vi "Lab Panel V5.12.vi"() -> ()   [LabVIEW 2013] (continued)
                      tunnel: w5308 -> [w5324 _]
                      tunnel: [w5323 FALSE] -> w5291
                      frame False {
                        n2899 = Equal?(x=w5325, y=w5324) -> (x = y?=w5323:bool)
                      }
                      frame True {
                      }
                    }
                    n2900 = Or(x=w5292, y=w5291) -> (x .or. y?=w5286:bool)
                    n2901 = Or(x=w5290, y=w5289) -> (x .or. y?=w5285:bool)
                    n2902 = Or(x=w5293, y=w5294) -> (x .or. y?=w5281:bool)
                    n2903 = Or(x=w5286, y=w5285) -> (x .or. y?=w5284:bool)
                    n2904 = Or(x=w5283, y=w5284) -> (x .or. y?=w5282:bool)
                    n2905 = Or(x=w5282, y=w5281) -> (x .or. y?=w5280:bool)
                  }
                  frame #3 {
                    n2906 = local read "on loops"() -> (w5363:dbl)
                    n2907 = local read "jig cycle"() -> (w5360:dbl)
                    n2908 = local read "Send Mail Now"() -> (w5354:bool)
                    n2909 = Add(x=w5363, y=3.0) -> (x+y=w5361:dbl)
                    n2910 = Equal?(x=w5360, y=w5361) -> (x = y?=w5355:bool)
                    n2911 = And(x=w5355, y=w5354) -> (x .and. y?=w5353:bool)
                    n2912 = And(x=w5359, y=w5355) -> (x .and. y?=w5358:bool)
                    n2913 = And(x=w5358, y=w5357) -> (x .and. y?=w5356:bool)
                    n2914 = Or(x=w5356, y=w5353) -> (x .or. y?=w5352:bool)
                    n2915 = case shown="True" w5352 {
                      tunnel: w5368 -> [_ w5374]
                      tunnel: w5367 -> [_ w5373]
                      tunnel: "Lab Panel Test Status" -> [_ w5372]
                      tunnel: w5365 -> [_ w5371]
                      tunnel: w5364 -> [_ w5370]
                      tunnel: w5351 -> [_ w5369]
                      frame False {
                      }
                      frame True {
                        n2916 = stacked-sequence {
                          tunnel: w5374 -> [w5382 _]
                          tunnel: w5373 -> [w5381 _]
                          tunnel: w5372 -> [w5380 _]
                          tunnel: w5371 -> [w5379 _]
                          tunnel: w5370 -> [w5378 _]
                          tunnel: w5369 -> [w5377 _]
                          frame #0 {
                            n2917 = call "sub vi - send mail v5.vi"("TO:"=w5382, "subject"=w5380, "from"=w5378, "out going server"=w5379, "message"=w5381) -> ("error out"=w5376:errorcluster)  [unwired: 10 in]
                            n2918 = Bundle(cluster=w5377, "mail error"=w5376) -> (w5375:T7)  [unwired: 6 in]
                            n2919 = local write "MAIL SETTINGS"(w5375) -> ()
                          }
                          frame #1 {
                            n2920 = local write "mail control"("") -> ()
                            n2921 = local write "Send Mail Now"(FALSE) -> ()
                          }
                        }
                      }
                    }
                  }
                }
              }
            }
          }
          frame #18 {
            # "save jig cycle values once all run switches are off"
            n2922 = stacked-sequence {
              tunnel: w5394 -> [_ w5423]
              tunnel: w5393 -> [_ w5422]
              tunnel: w5392 -> [_ w5421]
              tunnel: w5391 -> [_ w5420]
              tunnel: w5390 -> [_ w5419]
              tunnel: w5389 -> [_ w5418]
              tunnel: w5388 -> [_ w5417]
              tunnel: w5387 -> [_ w5416]
              tunnel: w5386 -> [_ w5415]
              tunnel: w5385 -> [_ w5414]
              frame #0 {
              }
              frame #1 {
                n2923 = Not(x=w5414) -> (.not. x?=w5397:bool)
                n2924 = Not(x=w5422) -> (.not. x?=w5412:bool)
                n2925 = Not(x=w5419) -> (.not. x?=w5407:bool)
                n2926 = Not(x=w5417) -> (.not. x?=w5403:bool)
                n2927 = Not(x=w5415) -> (.not. x?=w5399:bool)
                n2928 = Not(x=w5423) -> (.not. x?=w5413:bool)
                n2929 = Not(x=w5421) -> (.not. x?=w5411:bool)
                n2930 = Not(x=w5418) -> (.not. x?=w5405:bool)
                n2931 = Not(x=w5420) -> (.not. x?=w5409:bool)
                n2932 = Not(x=w5416) -> (.not. x?=w5401:bool)
                n2933 = local read "Save JC"() -> (w5425:bool)
                n2934 = And(x=w5413, y=w5412) -> (x .and. y?=w5410:bool)
                n2935 = And(x=w5410, y=w5411) -> (x .and. y?=w5408:bool)
                n2936 = And(x=w5408, y=w5409) -> (x .and. y?=w5406:bool)
                n2937 = And(x=w5406, y=w5407) -> (x .and. y?=w5404:bool)
                n2938 = And(x=w5404, y=w5405) -> (x .and. y?=w5402:bool)
                n2939 = And(x=w5402, y=w5403) -> (x .and. y?=w5400:bool)
                n2940 = And(x=w5400, y=w5401) -> (x .and. y?=w5398:bool)
                n2941 = And(x=w5398, y=w5399) -> (x .and. y?=w5396:bool)
                n2942 = And(x=w5396, y=w5397) -> (x .and. y?=w5395:bool)
                n2943 = And(x=w5395, y=w5425) -> (x .and. y?=w5424:bool)
                n2944 = case shown="True" w5424 {
                  tunnel: w5395 -> [w5426 _]
                  frame False {
                    n2945 = case shown="False" w5426 {
                      frame False {
                        n2946 = local write "Save JC"(TRUE) -> ()
                      }
                      frame True {
                      }
                    }
                  }
                  frame True {
                    n2947 = stacked-sequence {
                      frame #0 {
                        n2948 = String To Path(string="c:\\crabtree\\Jig Cycles\\") -> (path=w5438:path)
                        n2949 = Build Path(base path=w5438, name or relative path="jigcycles.bin") -> (appended path=w5436:path)
                        n2950 = Create Folder(path (use dialog)=w5438) -> (error out=w5440:errorcluster)  [unwired: 2 in, 2 out]
                        n2951 = local read "JIG RELAY CYCLES"() -> (w5430:T8)
                        n2952 = call <vilib>:"Clear Errors.vi"("error in (no error)"=w5440) -> ()  [unwired: 6 in, 1 out]
                        n2953 = local write "Save JC"(FALSE) -> ()
                        n2954 = Open/Create/Replace File(file path (use dialog)=w5436, operation (0:open)=T21."replace or create") -> (refnum out=w5434:refnum<file>, error out=w5435:errorcluster)  [unwired: 4 in, 1 out]
                        n2955 = Write to Binary File(file (use dialog)=w5434, data=w5430, error in=w5435) -> (refnum out=w5433:refnum<file>, error out=w5432:errorcluster)  [unwired: 3 in, 1 out]
                        n2956 = Close File(refnum=w5433, error in=w5432) -> (error out=w5431:errorcluster)  [unwired: 1 out]
                        n2957 = local write "data file error"(w5431) -> ()
                      }
                      frame #1 {
                        n2958 = local read "JIG RELAY CYCLES"() -> (w5463:T8)
                        n2959 = Unbundle By Name(w5463) -> ("LAB01-1"=w5458:dbl, "LAB01-2"=w5457:dbl, "LAB02-1"=w5455:dbl, "LAB02-2"=w5454:dbl, "LAB03-1"=w5452:dbl, "LAB03-2"=w5449:dbl, "LAB04-1"=w5448:dbl, "LAB04-2"=w5446:dbl, "LAB05-1"=w5444:dbl, "LAB05-2"=w5442:dbl)
                        n2960 = stacked-sequence {
                          tunnel: w5458 -> [w5466 _ _ _ _ _ _ _ _ _]
                          tunnel: 1000000 -> [w5469 w5479 w5489 w5499 w5509 w5519 w5529 w5539 w5549 w5559]
                          tunnel: [w5467 _ _ _ _ _ _ _ _ _] -> w5461
                          tunnel: "TEST STATION HAS REACHED 1 MILLION CYCLES, REPLACE  CONTROL RELAYS" -> [w5465 w5477 w5487 w5497 w5507 w5517 w5527 w5537 w5547 w5557]
                          tunnel: [_ w5476 _ _ _ _ _ _ _ _] -> w5459
                          tunnel: w5457 -> [_ w5475 _ _ _ _ _ _ _ _]
                          tunnel: [_ _ w5486 _ _ _ _ _ _ _] -> w5456
                          tunnel: w5455 -> [_ _ w5485 _ _ _ _ _ _ _]
                          tunnel: w5454 -> [_ _ _ w5496 _ _ _ _ _ _]
                          tunnel: [_ _ _ w5495 _ _ _ _ _ _] -> w5453
                          tunnel: w5452 -> [_ _ _ _ w5506 _ _ _ _ _]
                          tunnel: [_ _ _ _ w5505 _ _ _ _ _] -> w5451
                          tunnel: [_ _ _ _ _ w5516 _ _ _ _] -> w5450
                          tunnel: w5449 -> [_ _ _ _ _ w5515 _ _ _ _]
                          tunnel: w5448 -> [_ _ _ _ _ _ w5526 _ _ _]
                          tunnel: [_ _ _ _ _ _ w5525 _ _ _] -> w5447
                          tunnel: w5446 -> [_ _ _ _ _ _ _ w5536 _ _]
                          tunnel: [_ _ _ _ _ _ _ w5535 _ _] -> w5445
                          tunnel: w5444 -> [_ _ _ _ _ _ _ _ w5546 _]
                          tunnel: [_ _ _ _ _ _ _ _ w5545 _] -> w5443
                          tunnel: w5442 -> [_ _ _ _ _ _ _ _ _ w5556]
                          tunnel: [_ _ _ _ _ _ _ _ _ w5555] -> w5441
                          frame #0 {
                            n2961 = Greater?(x=w5466, y=w5469) -> (0:w5468:bool)
                            n2962 = case shown="True" w5468 {
                              tunnel: [w5470 0] -> w5467
                              tunnel: w5466 -> [w5470 _]
                              tunnel: w5465 -> [_ w5471]
                              frame False {
                              }
                              frame True {
                                n2963 = Concatenate Strings("LA01-1 ", w5471) -> (w5474:string)
                                n2964 = One Button Dialog(message=w5474) -> ()  [unwired: 1 in, 1 out]
                              }
                            }
                          }
                          frame #1 {
                            n2965 = Greater?(x=w5475, y=w5479) -> (0:w5478:bool)
                            n2966 = case shown="True" w5478 {
                              tunnel: [w5480 0] -> w5476
                              tunnel: w5475 -> [w5480 _]
                              tunnel: w5477 -> [_ w5481]
                              frame False {
                              }
                              frame True {
                                n2967 = Concatenate Strings("LA01-2 ", w5481) -> (w5484:string)
                                n2968 = One Button Dialog(message=w5484) -> ()  [unwired: 1 in, 1 out]
                              }
                            }
                          }
                          frame #2 {
                            n2969 = Greater?(x=w5485, y=w5489) -> (0:w5488:bool)
                            n2970 = case shown="True" w5488 {
                              tunnel: [w5490 0] -> w5486
                              tunnel: w5485 -> [w5490 _]
                              tunnel: w5487 -> [_ w5491]
                              frame False {
                              }
                              frame True {
                                n2971 = Concatenate Strings("LA02-1 ", w5491) -> (w5494:string)
                                n2972 = One Button Dialog(message=w5494) -> ()  [unwired: 1 in, 1 out]
                              }
                            }
                          }
                          frame #3 {
                            n2973 = Greater?(x=w5496, y=w5499) -> (0:w5498:bool)
                            n2974 = case shown="True" w5498 {
                              tunnel: [w5500 0] -> w5495
                              tunnel: w5496 -> [w5500 _]
                              tunnel: w5497 -> [_ w5501]
                              frame False {
                              }
                              frame True {
                                n2975 = Concatenate Strings("LA02-2 ", w5501) -> (w5504:string)
                                n2976 = One Button Dialog(message=w5504) -> ()  [unwired: 1 in, 1 out]
                              }
                            }
                          }
                          frame #4 {
                            n2977 = Greater?(x=w5506, y=w5509) -> (0:w5508:bool)
                            n2978 = case shown="True" w5508 {
                              tunnel: [w5510 0] -> w5505
                              tunnel: w5506 -> [w5510 _]
                              tunnel: w5507 -> [_ w5511]
                              frame False {
                              }
                              frame True {
                                n2979 = Concatenate Strings("LA03-1 ", w5511) -> (w5514:string)
                                n2980 = One Button Dialog(message=w5514) -> ()  [unwired: 1 in, 1 out]
                              }
                            }
                          }
                          frame #5 {
                            n2981 = Greater?(x=w5515, y=w5519) -> (0:w5518:bool)
                            n2982 = case shown="True" w5518 {
                              tunnel: [w5520 0] -> w5516
                              tunnel: w5515 -> [w5520 _]
                              tunnel: w5517 -> [_ w5521]
                              frame False {
                              }
                              frame True {
                                n2983 = Concatenate Strings("LA03-2 ", w5521) -> (w5524:string)
                                n2984 = One Button Dialog(message=w5524) -> ()  [unwired: 1 in, 1 out]
                              }
                            }
                          }
                          frame #6 {
                            n2985 = Greater?(x=w5526, y=w5529) -> (0:w5528:bool)
                            n2986 = case shown="True" w5528 {
                              tunnel: [w5530 0] -> w5525
                              tunnel: w5526 -> [w5530 _]
                              tunnel: w5527 -> [_ w5531]
                              frame False {
                              }
                              frame True {
                                n2987 = Concatenate Strings("LA04-1 ", w5531) -> (w5534:string)
                                n2988 = One Button Dialog(message=w5534) -> ()  [unwired: 1 in, 1 out]
                              }
                            }
                          }
                          frame #7 {
                            n2989 = Greater?(x=w5536, y=w5539) -> (0:w5538:bool)
                            n2990 = case shown="True" w5538 {
                              tunnel: [w5540 0] -> w5535
                              tunnel: w5536 -> [w5540 _]
                              tunnel: w5537 -> [_ w5541]
                              frame False {
                              }
                              frame True {
                                n2991 = Concatenate Strings("LA04-2 ", w5541) -> (w5544:string)
                                n2992 = One Button Dialog(message=w5544) -> ()  [unwired: 1 in, 1 out]
                              }
                            }
                          }
                          frame #8 {
                            n2993 = Greater?(x=w5546, y=w5549) -> (0:w5548:bool)
                            n2994 = case shown="True" w5548 {
                              tunnel: [w5550 0] -> w5545
                              tunnel: w5546 -> [w5550 _]
                              tunnel: w5547 -> [_ w5551]
                              frame False {
                              }
                              frame True {
                                n2995 = Concatenate Strings("LA05-1 ", w5551) -> (w5554:string)
                                n2996 = One Button Dialog(message=w5554) -> ()  [unwired: 1 in, 1 out]
                              }
                            }
                          }
                          frame #9 {
                            n2997 = Greater?(x=w5556, y=w5559) -> (0:w5558:bool)
                            n2998 = case shown="True" w5558 {
                              tunnel: [w5560 0] -> w5555
                              tunnel: w5556 -> [w5560 _]
                              tunnel: w5557 -> [_ w5561]
                              frame False {
                              }
                              frame True {
                                n2999 = Concatenate Strings("LA05-2 ", w5561) -> (w5564:string)
                                n3000 = One Button Dialog(message=w5564) -> ()  [unwired: 1 in, 1 out]
                              }
                            }
                          }
                        }
                        n3001 = Bundle By Name(cluster=w5463, "LAB01-1"=w5461, "LAB01-2"=w5459, "LAB02-1"=w5456, "LAB02-2"=w5453, "LAB03-1"=w5451, "LAB03-2"=w5450, "LAB04-1"=w5447, "LAB04-2"=w5445, "LAB05-1"=w5443, "LAB05-2"=w5441) -> (w5462:T8)
                        n3002 = local write "JIG RELAY CYCLES"(w5462) -> ()
                      }
                    }
                  }
                }
              }
            }
          }
          frame #19 {
            # "get temperature values"
            n3003 = local read "Panel #"() -> (w5565:dbl)
            n3004 = local read "Simulate"() -> (w5578:bool)
            n3005 = local read "Temp Test Cal"() -> (w5575:dbl)
            n3006 = stacked-sequence {
              seq-local: [w5581 _] -> [_ w5624]
              tunnel: w5578 -> [_ w5638]
              tunnel: T14 {"1  (A) cal"=1.0, "1 (V) cal"=1.0, "1 (PF) cal"=1.0, "1 (TL) cal"=1.0, "1 (TN) cal"=1.0, "2 (A) cal"=1.0, "2 (V) cal"=1.0, "2 (PF) cal"=1.0, "2 (TL) cal"=1.0, "2 (TN) cal"=1.0} ("CAL LAB01") -> [_ w5637]
              tunnel: w5576 -> [_ w5636]
              tunnel: w5575 -> [_ w5635]
              tunnel: w5574 -> [_ w5634]
              tunnel: w5573 -> [_ w5633]
              tunnel: w5572 -> [_ w5632]
              tunnel: w5571 -> [_ w5631]
              tunnel: w5570 -> [_ w5630]
              tunnel: w5569 -> [_ w5629]
              tunnel: w5568 -> [_ w5628]
              tunnel: w5567 -> [_ w5627]
              tunnel: w5566 -> [_ w5626]
              tunnel: w5565 -> [_ w5625]
              frame #0 {
                n3007 = local read "Select COM port"() -> (w5582:refnum<visa-resource-name>)
                "COM port" <- w5582
                n3008 = global write "Global 1.vi" "COM port"(w5582) -> ()
                n3009 = global write "Global 1.vi" "tmp dly lps"("Temp Delay Lps") -> ()
                n3010 = global write "Global 1.vi" "dly value"("Temp Value") -> ()
                n3011 = local read "jig cycle"() -> (w5584:dbl)
                n3012 = local read "on loops"() -> (w5586:dbl)
                n3013 = Add(x=w5586, y=3) -> (x+y=w5587:dbl)
                n3014 = local read "Panel #"() -> (w5583:dbl)
                n3015 = Equal?(x=w5584, y=w5587) -> (x = y?=w5581:bool)
                n3016 = case shown="True" w5581 {
                  tunnel: w5583 -> [_ w5592]
                  frame False {
                  }
                  frame True {
                    n3017 = local read "Simulate"() -> (w5589:bool)
                    n3018 = case shown="1" w5592 {
                      tunnel: 1.0 -> [_ w5599 w5602 w5609 w5614 w5620]
                      tunnel: w5589 -> [_ w5595 w5601 w5607 w5615 w5619]
                      tunnel: [FALSE w5594 w5600 w5606 w5612 w5618] -> w5588
                      frame 0, Default {
                      }
                      frame 1 {
                        w5597 = FALSE
                        n3019 = call "sub vi - GET ALL TEMP v7.vi"("LA01-EN"=TRUE, "simulate"=w5595, "LA02-EN"=w5597, "LA03-EN"=w5597, "LA04-EN"=w5597, "LA05-EN"=w5597, "Gen Cal Value"=w5599) -> ("LA01 TEMP"=w5596:T24, "error"=w5594:bool)  [unwired: 3 in, 4 out]
                        n3020 = local write "LAB01 TEMP"(w5596) -> ()
                      }
                      frame 2 {
                        w5603 = FALSE
                        n3021 = call "sub vi - GET ALL TEMP v7.vi"("LA01-EN"=w5603, "simulate"=w5601, "LA02-EN"=TRUE, "LA03-EN"=w5603, "LA04-EN"=w5603, "LA05-EN"=w5603, "Gen Cal Value"=w5602) -> ("LA02 TEMP"=w5605:T24, "error"=w5600:bool)  [unwired: 3 in, 4 out]
                        n3022 = local write "LAB02 TEMP"(w5605) -> ()
                      }
                      frame 3 {
                        w5610 = FALSE
                        n3023 = call "sub vi - GET ALL TEMP v7.vi"("LA01-EN"=w5610, "simulate"=w5607, "LA02-EN"=w5610, "LA03-EN"=TRUE, "LA04-EN"=w5610, "LA05-EN"=w5610, "Gen Cal Value"=w5609) -> ("LA03 TEMP"=w5608:T24, "error"=w5606:bool)  [unwired: 3 in, 4 out]
                        n3024 = local write "LAB03 TEMP"(w5608) -> ()
                      }
                      frame 4 {
                        w5616 = FALSE
                        n3025 = call "sub vi - GET ALL TEMP v7.vi"("LA01-EN"=w5616, "simulate"=w5615, "LA02-EN"=w5616, "LA03-EN"=w5616, "LA04-EN"=TRUE, "LA05-EN"=w5616, "Gen Cal Value"=w5614) -> ("LA04 TEMP"=w5613:T24, "error"=w5612:bool)  [unwired: 3 in, 4 out]
                        n3026 = local write "LAB04 TEMP"(w5613) -> ()
                      }
                      frame 5 {
                        w5622 = FALSE
                        n3027 = call "sub vi - GET ALL TEMP v7.vi"("LA01-EN"=w5622, "simulate"=w5619, "LA02-EN"=w5622, "LA03-EN"=w5622, "LA04-EN"=w5622, "LA05-EN"=TRUE, "Gen Cal Value"=w5620) -> ("error"=w5618:bool, "LA05 TEMP"=w5621:T24)  [unwired: 3 in, 4 out]
                        n3028 = local write "LAB05 TEMP"(w5621) -> ()
                      }
                    }
                    "Error Temp" <- w5588
                    n3029 = local write "TEMP"(TRUE) -> ()
                  }
                }
              }
              frame #1 {
                n3030 = case shown="True" w5624 {
                  tunnel: w5638 -> [_ w5652]
                  tunnel: w5637 -> [_ w5651]
                  tunnel: w5636 -> [_ w5650]
                  tunnel: w5635 -> [_ w5649]
                  tunnel: w5634 -> [_ w5648]
                  tunnel: w5633 -> [_ w5647]
                  tunnel: w5632 -> [_ w5646]
                  tunnel: w5631 -> [_ w5645]
                  tunnel: w5630 -> [_ w5644]
                  tunnel: w5629 -> [_ w5643]
                  tunnel: w5628 -> [_ w5642]
                  tunnel: w5627 -> [_ w5641]
                  tunnel: w5626 -> [_ w5640]
                  tunnel: w5625 -> [_ w5639]
                  frame False {
                  }
                  frame True {
                    n3031 = case shown="1" w5639 {
                      tunnel: w5652 -> [_ w5665 w5710 w5755 w5800 w5845]
                      tunnel: w5651 -> [_ w5664 w5709 w5754 w5799 w5844]
                      tunnel: w5650 -> [_ w5654 _ _ _ _]
                      tunnel: w5649 -> [_ w5659 w5708 w5753 w5798 w5843]
                      tunnel: w5648 -> [_ w5653 _ _ _ _]
                      tunnel: w5647 -> [_ _ w5699 _ _ _]
                      tunnel: w5646 -> [_ _ w5698 _ _ _]
                      tunnel: w5645 -> [_ _ _ w5744 _ _]
                      tunnel: w5644 -> [_ _ _ w5743 _ _]
                      tunnel: w5643 -> [_ _ _ _ w5789 _]
                      tunnel: w5642 -> [_ _ _ _ w5788 _]
                      tunnel: w5641 -> [_ _ _ _ _ w5834]
                      tunnel: w5640 -> [_ _ _ _ _ w5833]
                      frame ..0 {
                      }
                      frame 1 {
                        n3032 = case shown="False" w5665 {
                          tunnel: [w5696 w5697] -> w5681
                          tunnel: w5664 -> [_ w5697]
                          frame False {
                            n3033 = local read "CAL LAB01"() -> (w5696:T14)
                          }
                          frame True {
                          }
                        }
                        n3034 = local read "TEMP LA01"() -> (w5672:T9)
                        n3035 = local read "LAB01 TEMP"() -> (w5671:T12)
                        n3036 = call "sub vi - temperature delay v3.vi"("2-run"=w5653, "1-run"=w5654, "temp values IN"=w5672, "temp signals"=w5671) -> ("T2-N"=w5667:dbl, "T2-L"=w5668:dbl, "T1-N"=w5669:dbl, "T1-L"=w5670:dbl, "temp values OUT"=w5666:T43)  [unwired: 3 in]
                        n3037 = Unbundle By Name(w5681) -> ("1 (TL) cal"=w5676:dbl, "1 (TN) cal"=w5675:dbl, "2 (TL) cal"=w5674:dbl, "2 (TN) cal"=w5673:dbl)  [unwired: 6 out]
                        n3038 = local write "TEMP LA01"(w5666) -> ()
                        n3039 = Multiply(x=w5670, y=w5676) -> (x*y=w5663:dbl)
                        n3040 = Multiply(x=w5669, y=w5675) -> (x*y=w5661:dbl)
                        n3041 = Multiply(x=w5668, y=w5674) -> (x*y=w5658:dbl)
                        n3042 = Multiply(x=w5667, y=w5673) -> (x*y=w5657:dbl)
                        n3043 = case shown="True" w5654 {
                          tunnel: w5663 -> [w5690 w5695]
                          tunnel: w5659 -> [_ w5693]
                          tunnel: [w5690 w5694] -> w5662
                          tunnel: w5661 -> [w5689 w5692]
                          tunnel: [w5689 w5691] -> w5660
                          frame False {
                          }
                          frame True {
                            n3044 = Multiply(x=w5693, y=w5692) -> (x*y=w5691:dbl)
                            n3045 = Multiply(x=w5693, y=w5695) -> (x*y=w5694:dbl)
                          }
                        }
                        n3046 = case shown="True" w5653 {
                          tunnel: w5658 -> [w5683 w5688]
                          tunnel: w5659 -> [_ w5686]
                          tunnel: [w5683 w5687] -> w5656
                          tunnel: w5657 -> [w5682 w5685]
                          tunnel: [w5682 w5684] -> w5655
                          frame False {
                          }
                          frame True {
                            n3047 = Multiply(x=w5686, y=w5685) -> (x*y=w5684:dbl)
                            n3048 = Multiply(x=w5686, y=w5688) -> (x*y=w5687:dbl)
                          }
                        }
                        n3049 = local read "SIG LAB01-2"() -> (w5678:T2)
                        n3050 = local read "SIG LAB01-1"() -> (w5680:T2)
                        n3051 = Bundle By Name(cluster=w5680, "Tmp Live"=w5662, "Tmp Neut"=w5660) -> (w5679:T2)
                        n3052 = Bundle By Name(cluster=w5678, "Tmp Live"=w5656, "Tmp Neut"=w5655) -> (w5677:T2)
                        n3053 = local write "SIG LAB01-1"(w5679) -> ()
                        n3054 = local write "SIG LAB01-2"(w5677) -> ()
                      }
                      frame 2 {
                        n3055 = case shown="True" w5710 {
                          tunnel: [w5741 w5742] -> w5726
                          tunnel: w5709 -> [_ w5742]
                          frame False {
                            n3056 = local read "CAL LAB02"() -> (w5741:T15)
                          }
                          frame True {
                          }
                        }
                        n3057 = local read "LAB02 TEMP"() -> (w5717:T12)
                        n3058 = local read "TEMP LA02"() -> (w5716:T9)
                        n3059 = call "sub vi - temperature delay v3.vi"("2-run"=w5698, "1-run"=w5699, "temp values IN"=w5716, "temp signals"=w5717) -> ("T2-N"=w5711:dbl, "T2-L"=w5712:dbl, "T1-N"=w5713:dbl, "T1-L"=w5714:dbl, "temp values OUT"=w5715:T43)  [unwired: 3 in]
                        n3060 = Unbundle By Name(w5726) -> ("1 (TL) cal"=w5721:dbl, "1 (TN) cal"=w5720:dbl, "2 (TL) cal"=w5719:dbl, "2 (TN) cal"=w5718:dbl)  [unwired: 6 out]
                        n3061 = local write "TEMP LA02"(w5715) -> ()
                        n3062 = Multiply(x=w5714, y=w5721) -> (x*y=w5707:dbl)
                        n3063 = Multiply(x=w5713, y=w5720) -> (x*y=w5706:dbl)
                        n3064 = Multiply(x=w5712, y=w5719) -> (x*y=w5703:dbl)
                        n3065 = Multiply(x=w5711, y=w5718) -> (x*y=w5702:dbl)
                        n3066 = case shown="True" w5699 {
                          tunnel: w5707 -> [w5735 w5740]
                          tunnel: w5708 -> [_ w5738]
                          tunnel: [w5735 w5739] -> w5705
                          tunnel: w5706 -> [w5734 w5737]
                          tunnel: [w5734 w5736] -> w5704
                          frame False {
                          }
                          frame True {
                            n3067 = Multiply(x=w5738, y=w5737) -> (x*y=w5736:dbl)
                            n3068 = Multiply(x=w5738, y=w5740) -> (x*y=w5739:dbl)
                          }
                        }
                        n3069 = case shown="True" w5698 {
                          tunnel: w5703 -> [w5728 w5733]
                          tunnel: w5708 -> [_ w5731]
                          tunnel: [w5728 w5732] -> w5701
                          tunnel: w5702 -> [w5727 w5730]
                          tunnel: [w5727 w5729] -> w5700
                          frame False {
                          }
                          frame True {
                            n3070 = Multiply(x=w5731, y=w5730) -> (x*y=w5729:dbl)
                            n3071 = Multiply(x=w5731, y=w5733) -> (x*y=w5732:dbl)
                          }
                        }
                        n3072 = local read "SIG LAB02-2"() -> (w5723:T2)
                        n3073 = local read "SIG LAB02-1"() -> (w5725:T2)
                        n3074 = Bundle By Name(cluster=w5725, "Tmp Live"=w5705, "Tmp Neut"=w5704) -> (w5724:T2)
                        n3075 = Bundle By Name(cluster=w5723, "Tmp Live"=w5701, "Tmp Neut"=w5700) -> (w5722:T2)
                        n3076 = local write "SIG LAB02-1"(w5724) -> ()
                        n3077 = local write "SIG LAB02-2"(w5722) -> ()
                      }
                      frame 3 {
                        n3078 = case shown="False" w5755 {
                          tunnel: [w5786 w5787] -> w5771
                          tunnel: w5754 -> [_ w5787]
                          frame False {
                            n3079 = local read "CAL LAB03"() -> (w5786:T14)
                          }
                          frame True {
                          }
                        }
                        n3080 = local read "TEMP LA03"() -> (w5761:T9)
                        n3081 = local read "LAB03 TEMP"() -> (w5762:T12)
                        n3082 = call "sub vi - temperature delay v3.vi"("2-run"=w5743, "1-run"=w5744, "temp values IN"=w5761, "temp signals"=w5762) -> ("T2-N"=w5756:dbl, "T2-L"=w5757:dbl, "T1-N"=w5758:dbl, "T1-L"=w5759:dbl, "temp values OUT"=w5760:T43)  [unwired: 3 in]
                        n3083 = Unbundle By Name(w5771) -> ("1 (TL) cal"=w5766:dbl, "1 (TN) cal"=w5765:dbl, "2 (TL) cal"=w5764:dbl, "2 (TN) cal"=w5763:dbl)  [unwired: 6 out]
                        n3084 = local write "TEMP LA03"(w5760) -> ()
                        n3085 = Multiply(x=w5759, y=w5766) -> (x*y=w5752:dbl)
                        n3086 = Multiply(x=w5758, y=w5765) -> (x*y=w5751:dbl)
                        n3087 = Multiply(x=w5757, y=w5764) -> (x*y=w5748:dbl)
                        n3088 = Multiply(x=w5756, y=w5763) -> (x*y=w5747:dbl)
                        n3089 = case shown="True" w5743 {
                          tunnel: w5748 -> [w5773 w5778]
                          tunnel: w5753 -> [_ w5776]
                          tunnel: [w5773 w5777] -> w5746
                          tunnel: w5747 -> [w5772 w5775]
                          tunnel: [w5772 w5774] -> w5745
                          frame False {
                          }
                          frame True {
                            n3090 = Multiply(x=w5776, y=w5775) -> (x*y=w5774:dbl)
                            n3091 = Multiply(x=w5776, y=w5778) -> (x*y=w5777:dbl)
                          }
                        }
                        n3092 = case shown="True" w5744 {
                          tunnel: w5752 -> [w5780 w5785]
                          tunnel: w5753 -> [_ w5783]
                          tunnel: [w5780 w5784] -> w5750
                          tunnel: w5751 -> [w5779 w5782]
                          tunnel: [w5779 w5781] -> w5749
                          frame False {
                          }
                          frame True {
                            n3093 = Multiply(x=w5783, y=w5782) -> (x*y=w5781:dbl)
                            n3094 = Multiply(x=w5783, y=w5785) -> (x*y=w5784:dbl)
                          }
                        }
                        n3095 = local read "SIG LAB03-2"() -> (w5768:T2)
                        n3096 = local read "SIG LAB03-1"() -> (w5770:T2)
                        n3097 = Bundle By Name(cluster=w5770, "Tmp Live"=w5750, "Tmp Neut"=w5749) -> (w5769:T2)
                        n3098 = Bundle By Name(cluster=w5768, "Tmp Live"=w5746, "Tmp Neut"=w5745) -> (w5767:T2)
                        n3099 = local write "SIG LAB03-1"(w5769) -> ()
                        n3100 = local write "SIG LAB03-2"(w5767) -> ()
                      }
                      frame 4 {
                        n3101 = case shown="False" w5800 {
                          tunnel: [w5831 w5832] -> w5816
                          tunnel: w5799 -> [_ w5832]
                          frame False {
                            n3102 = local read "CAL LAB04"() -> (w5831:T14)
                          }
                          frame True {
                          }
                        }
                        n3103 = local read "LAB04 TEMP"() -> (w5806:T12)
                        n3104 = local read "TEMP LA04"() -> (w5807:T9)
                        n3105 = call "sub vi - temperature delay v3.vi"("2-run"=w5788, "1-run"=w5789, "temp values IN"=w5807, "temp signals"=w5806) -> ("T2-N"=w5801:dbl, "T2-L"=w5802:dbl, "T1-N"=w5803:dbl, "T1-L"=w5804:dbl, "temp values OUT"=w5805:T43)  [unwired: 3 in]
                        n3106 = Unbundle By Name(w5816) -> ("1 (TL) cal"=w5811:dbl, "1 (TN) cal"=w5810:dbl, "2 (TL) cal"=w5809:dbl, "2 (TN) cal"=w5808:dbl)  [unwired: 6 out]
                        n3107 = local write "TEMP LA04"(w5805) -> ()
                        n3108 = Multiply(x=w5804, y=w5811) -> (x*y=w5797:dbl)
                        n3109 = Multiply(x=w5803, y=w5810) -> (x*y=w5796:dbl)
                        n3110 = Multiply(x=w5802, y=w5809) -> (x*y=w5793:dbl)
                        n3111 = Multiply(x=w5801, y=w5808) -> (x*y=w5792:dbl)
                        n3112 = case shown="True" w5788 {
                          tunnel: w5793 -> [w5818 w5823]
                          tunnel: w5798 -> [_ w5821]
                          tunnel: [w5818 w5822] -> w5791
                          tunnel: w5792 -> [w5817 w5820]
                          tunnel: [w5817 w5819] -> w5790
                          frame False {
                          }
                          frame True {
                            n3113 = Multiply(x=w5821, y=w5820) -> (x*y=w5819:dbl)
                            n3114 = Multiply(x=w5821, y=w5823) -> (x*y=w5822:dbl)
                          }
                        }
                        n3115 = case shown="True" w5789 {
                          tunnel: w5797 -> [w5825 w5830]
                          tunnel: w5798 -> [_ w5828]
                          tunnel: [w5825 w5829] -> w5795
                          tunnel: w5796 -> [w5824 w5827]
                          tunnel: [w5824 w5826] -> w5794
                          frame False {
                          }
                          frame True {
                            n3116 = Multiply(x=w5828, y=w5827) -> (x*y=w5826:dbl)
                            n3117 = Multiply(x=w5828, y=w5830) -> (x*y=w5829:dbl)
                          }
                        }
                        n3118 = local read "SIG LAB04-2"() -> (w5813:T2)
                        n3119 = local read "SIG LAB04-1"() -> (w5815:T2)
                        n3120 = Bundle By Name(cluster=w5815, "Tmp Live"=w5795, "Tmp Neut"=w5794) -> (w5814:T2)
                        n3121 = Bundle By Name(cluster=w5813, "Tmp Live"=w5791, "Tmp Neut"=w5790) -> (w5812:T2)
                        n3122 = local write "SIG LAB04-1"(w5814) -> ()
                        n3123 = local write "SIG LAB04-2"(w5812) -> ()
                      }
                      frame 5.. {
                        n3124 = case shown="False" w5845 {
                          tunnel: [w5876 w5877] -> w5861
                          tunnel: w5844 -> [_ w5877]
                          frame False {
                            n3125 = local read "CAL LAB05"() -> (w5876:T14)
                          }
                          frame True {
                          }
                        }
                        n3126 = local read "LAB05 TEMP"() -> (w5851:T12)
                        n3127 = local read "TEMP LA05"() -> (w5852:T9)
                        n3128 = call "sub vi - temperature delay v3.vi"("2-run"=w5833, "1-run"=w5834, "temp values IN"=w5852, "temp signals"=w5851) -> ("T2-N"=w5847:dbl, "T2-L"=w5848:dbl, "T1-N"=w5849:dbl, "T1-L"=w5850:dbl, "temp values OUT"=w5846:T43)  [unwired: 3 in]
                        n3129 = local write "TEMP LA05"(w5846) -> ()
                        n3130 = Unbundle By Name(w5861) -> ("1 (TL) cal"=w5853:dbl, "1 (TN) cal"=w5856:dbl, "2 (TL) cal"=w5855:dbl, "2 (TN) cal"=w5854:dbl)  [unwired: 6 out]
                        n3131 = Multiply(x=w5850, y=w5853) -> (x*y=w5842:dbl)
                        n3132 = Multiply(x=w5849, y=w5856) -> (x*y=w5841:dbl)
                        n3133 = Multiply(x=w5848, y=w5855) -> (x*y=w5838:dbl)
                        n3134 = Multiply(x=w5847, y=w5854) -> (x*y=w5837:dbl)
                        n3135 = case shown="True" w5833 {
                          tunnel: w5838 -> [w5863 w5868]
                          tunnel: w5843 -> [_ w5866]
                          tunnel: [w5863 w5867] -> w5836
                          tunnel: w5837 -> [w5862 w5865]
                          tunnel: [w5862 w5864] -> w5835
                          frame False {
                          }
                          frame True {
                            n3136 = Multiply(x=w5866, y=w5865) -> (x*y=w5864:dbl)
                            n3137 = Multiply(x=w5866, y=w5868) -> (x*y=w5867:dbl)
                          }
                        }
                        n3138 = case shown="True" w5834 {
                          tunnel: w5842 -> [w5870 w5875]
                          tunnel: w5843 -> [_ w5873]
                          tunnel: [w5870 w5874] -> w5840
                          tunnel: w5841 -> [w5869 w5872]
                          tunnel: [w5869 w5871] -> w5839
                          frame False {
                          }
                          frame True {
                            n3139 = Multiply(x=w5873, y=w5872) -> (x*y=w5871:dbl)
                            n3140 = Multiply(x=w5873, y=w5875) -> (x*y=w5874:dbl)
                          }
                        }
                        n3141 = local read "SIG LAB05-1"() -> (w5860:T2)
                        n3142 = Bundle By Name(cluster=w5860, "Tmp Live"=w5840, "Tmp Neut"=w5839) -> (w5859:T2)
                        n3143 = local read "SIG LAB05-2"() -> (w5858:T2)
                        n3144 = Bundle By Name(cluster=w5858, "Tmp Live"=w5836, "Tmp Neut"=w5835) -> (w5857:T2)
                        n3145 = local write "SIG LAB05-1"(w5859) -> ()
                        n3146 = local write "SIG LAB05-2"(w5857) -> ()
                      }
                    }
                  }
                }
              }
            }
          }
          frame #20 {
            # "write data to display panel"
            n3147 = global write "Global display 1.vi" "TEST 5-2"(w5912) -> ()
            n3148 = global write "Global display 1.vi" "TEST 4-2"(w5914) -> ()
            n3149 = global write "Global display 1.vi" "TEST 1-2"(w5920) -> ()
            n3150 = global write "Global display 1.vi" "TEST 3-1"(w5917) -> ()
            n3151 = global write "Global display 1.vi" "TEST 5-1"(w5913) -> ()
            n3152 = global write "Global display 1.vi" "TEST 1-1"(w5921) -> ()
            n3153 = global write "Global display 1.vi" "TEST 3-2"(w5916) -> ()
            n3154 = global write "Global display 1.vi" "TEST 4-1"(w5915) -> ()
            n3155 = global write "Global display 1.vi" "TEST 2-2"(w5918) -> ()
            n3156 = global write "Global display 1.vi" "TEST 2-1"(w5919) -> ()
            n3157 = global read "Global display 3.vi" "log 1-1"() -> (→"LOG LAB01-1":string)
            n3158 = global read "Global display 3.vi" "log 3-1"() -> (→"LOG LAB03-1":string)
            n3159 = global read "Global display 3.vi" "log 1-2"() -> (→"LOG LAB01-2":string)
            n3160 = property on="Tab Control 2" class="TabCtl (strict)"() -> ("Pages"=w5911:refnum<vi>[])  [unwired: 2 in, 2 out]
            n3161 = global read "Global display 3.vi" "log 2-1"() -> (→"LOG LAB02-1":string)
            n3162 = global read "Global display 3.vi" "log 2-2"() -> (→"LOG LAB02-2":string)
            n3163 = global read "Global display 3.vi" "log 4-2"() -> (→"LOG LAB04-2":string)
            n3164 = global read "Global display 3.vi" "log 5-2"() -> (→"LOG LAB05-2":string)
            n3165 = global read "Global display 3.vi" "log 5-1"() -> (→"LOG LAB05-1":string)
            n3166 = global read "Global display 3.vi" "log 4-1"() -> (→"LOG LAB04-1":string)
            n3167 = global read "Global display 3.vi" "log 3-2"() -> (→"LOG LAB03-2":string)
            n3168 = Index Array(array=w5911, index=8) -> (element=w5909:refnum<vi>)
            n3169 = property class="Page"(reference=w5909) -> ("PageVis"=w5908:bool)  [unwired: 1 in, 2 out]
            n3170 = global write "Global display 3.vi" "admin"(w5908) -> ()
            n3171 = local read "O/I  LAB05-2"() -> (w5962:bool)
            n3172 = local read "O/I  LAB05-1"() -> (w5963:bool)
            n3173 = local read "O/I  LAB03-2"() -> (w5966:bool)
            n3174 = local read "O/I  LAB04-2"() -> (w5964:bool)
            n3175 = local read "O/I  LAB04-1"() -> (w5965:bool)
            n3176 = local read "O/I  LAB03-1"() -> (w5967:bool)
            n3177 = local read "O/I  LAB01-2"() -> (w5970:bool)
            n3178 = local read "O/I  LAB01-1"() -> (w5971:bool)
            n3179 = local read "O/I  LAB02-1"() -> (w5969:bool)
            n3180 = local read "O/I  LAB02-2"() -> (w5968:bool)
            n3181 = global write "Global display 1.vi" "5-2 O/F"(w5962) -> ()
            n3182 = global write "Global display 1.vi" "5-1 O/F"(w5963) -> ()
            n3183 = global write "Global display 1.vi" "4-1 O/F"(w5965) -> ()
            n3184 = global write "Global display 1.vi" "4-2 O/F"(w5964) -> ()
            n3185 = global write "Global display 1.vi" "3-2 O/F"(w5966) -> ()
            n3186 = global write "Global display 1.vi" "3-1 O/F"(w5967) -> ()
            n3187 = global write "Global display 1.vi" "2-2 O/F"(w5968) -> ()
            n3188 = global write "Global display 1.vi" "2-1 O/F"(w5969) -> ()
            n3189 = global write "Global display 1.vi" "1-2 O/F"(w5970) -> ()
            n3190 = global write "Global display 1.vi" "1-1 O/F"(w5971) -> ()
            n3191 = local read "TEMP START LAB02-2"() -> (w5894:cluster{"TL":dbl, "TN":dbl})
            n3192 = local read "run lab05-2"() -> (w5952:bool)
            n3193 = local read "TEMP START LAB01-2"() -> (w5896:cluster{"TL":dbl, "TN":dbl})
            n3194 = local read "TEMP START LAB02-1"() -> (w5895:cluster{"TL":dbl, "TN":dbl})
            n3195 = local read "TEMP START LAB04-1"() -> (w5891:cluster{"TL":dbl, "TN":dbl})
            n3196 = local read "TEMP START LAB04-2"() -> (w5890:cluster{"TL":dbl, "TN":dbl})
            n3197 = local read "run lab04-1"() -> (w5955:bool)
            n3198 = local read "run lab04-2"() -> (w5954:bool)
            n3199 = local read "run lab05-1"() -> (w5953:bool)
            n3200 = local read "TEMP START LAB01-1"() -> (w5897:cluster{"TL":dbl, "TN":dbl})
            n3201 = local read "TEMP START LAB05-2"() -> (w5888:cluster{"TL":dbl, "TN":dbl})
            n3202 = local read "TEMP START LAB05-1"() -> (w5889:cluster{"TL":dbl, "TN":dbl})
            n3203 = local read "run lab03-2"() -> (w5956:bool)
            n3204 = local read "TEMP START LAB03-2"() -> (w5892:cluster{"TL":dbl, "TN":dbl})
            n3205 = local read "TEMP START LAB03-1"() -> (w5893:cluster{"TL":dbl, "TN":dbl})
            n3206 = local read "run lab02-1"() -> (w5959:bool)
            n3207 = local read "run lab03-1"() -> (w5957:bool)
            n3208 = local read "run lab01-2"() -> (w5960:bool)
            n3209 = local read "run lab02-2"() -> (w5958:bool)
            n3210 = local read "run lab01-1"() -> (w5961:bool)
            n3211 = global write "Global display 1.vi" "5-2 R/S"(w5952) -> ()
            n3212 = global write "Global display 1.vi" "5-1 R/S"(w5953) -> ()
            n3213 = global write "Global display 1.vi" "4-2 R/S"(w5954) -> ()
            n3214 = global write "Global display 1.vi" "4-1 R/S"(w5955) -> ()
            n3215 = global write "Global display 1.vi" "3-2 R/S"(w5956) -> ()
            n3216 = global write "Global display 1.vi" "1-2 R/S"(w5960) -> ()
            n3217 = global write "Global display 1.vi" "2-1 R/S"(w5959) -> ()
            n3218 = global write "Global display 1.vi" "3-1 R/S"(w5957) -> ()
            n3219 = global write "Global display 1.vi" "2-2 R/S"(w5958) -> ()
            n3220 = global write "Global display 1.vi" "1-1 R/S"(w5961) -> ()
            n3221 = global write "Global display 3.vi" "TEMP ST 05-2"(w5888) -> ()
            n3222 = global write "Global display 3.vi" "TEMP ST 05-1"(w5889) -> ()
            n3223 = global write "Global display 3.vi" "TEMP ST 03-2"(w5892) -> ()
            n3224 = global write "Global display 3.vi" "TEMP ST 04-2"(w5890) -> ()
            n3225 = global write "Global display 3.vi" "TEMP ST 01-1"(w5897) -> ()
            n3226 = global write "Global display 3.vi" "TEMP ST 01-2"(w5896) -> ()
            n3227 = global write "Global display 3.vi" "TEMP ST 04-1"(w5891) -> ()
            n3228 = global write "Global display 3.vi" "TEMP ST 02-1"(w5895) -> ()
            n3229 = global write "Global display 3.vi" "TEMP ST 02-2"(w5894) -> ()
            n3230 = global write "Global display 3.vi" "TEMP ST 03-1"(w5893) -> ()
            n3231 = local read "DISP LAB04-2"() -> (w5944:T4)
            n3232 = local read "DISP LAB05-1"() -> (w5943:T4)
            n3233 = local read "DISP LAB04-1"() -> (w5945:T4)
            n3234 = local read "DISP LAB05-2"() -> (w5942:T4)
            n3235 = local read "DISP LAB03-1"() -> (w5947:T4)
            n3236 = local read "DISP LAB03-2"() -> (w5946:T4)
            n3237 = local read "DISP LAB01-2"() -> (w5950:T4)
            n3238 = local read "DISP LAB02-1"() -> (w5949:T4)
            n3239 = local read "DISP LAB02-2"() -> (w5948:T4)
            n3240 = local read "DISP LAB01-1"() -> (w5951:T4)
            n3241 = local read "TEMP RISE LAB05-1"() -> (w5879:cluster{"TL":dbl, "TN":dbl})
            n3242 = local read "TEMP RISE LAB05-2"() -> (w5878:cluster{"TL":dbl, "TN":dbl})
            n3243 = local read "TEMP RISE LAB04-2"() -> (w5880:cluster{"TL":dbl, "TN":dbl})
            n3244 = local read "TEMP RISE LAB04-1"() -> (w5881:cluster{"TL":dbl, "TN":dbl})
            n3245 = local read "TEMP RISE LAB03-2"() -> (w5882:cluster{"TL":dbl, "TN":dbl})
            n3246 = local read "TEMP RISE LAB03-1"() -> (w5883:cluster{"TL":dbl, "TN":dbl})
            n3247 = local read "TEMP RISE LAB01-2"() -> (w5886:cluster{"TL":dbl, "TN":dbl})
            n3248 = local read "TEMP RISE LAB02-2"() -> (w5884:cluster{"TL":dbl, "TN":dbl})
            n3249 = local read "TEMP RISE LAB01-1"() -> (w5887:cluster{"TL":dbl, "TN":dbl})
            n3250 = local read "TEMP RISE LAB02-1"() -> (w5885:cluster{"TL":dbl, "TN":dbl})
            n3251 = global write "Global display 2.vi" "DISP LAB05-1"(w5943) -> ()
            n3252 = global write "Global display 2.vi" "DISP LAB05-2"(w5942) -> ()
            n3253 = global write "Global display 2.vi" "DISP LAB04-2"(w5944) -> ()
            n3254 = global write "Global display 2.vi" "DISP LAB02-1"(w5949) -> ()
            n3255 = global write "Global display 2.vi" "DISP LAB02-2"(w5948) -> ()
            n3256 = global write "Global display 2.vi" "DISP LAB04-1"(w5945) -> ()
            n3257 = global write "Global display 2.vi" "DISP LAB01-2"(w5950) -> ()
            n3258 = global write "Global display 2.vi" "DISP LAB01-1"(w5951) -> ()
            n3259 = global write "Global display 2.vi" "DISP LAB03-1"(w5947) -> ()
            n3260 = global write "Global display 2.vi" "DISP LAB03-2"(w5946) -> ()
            n3261 = global write "Global display 3.vi" "TEMP RS 05-2"(w5878) -> ()
            n3262 = global write "Global display 3.vi" "TEMP RS 05-1"(w5879) -> ()
            n3263 = global write "Global display 3.vi" "TEMP RS 03-2"(w5882) -> ()
            n3264 = global write "Global display 3.vi" "TEMP RS 02-1"(w5885) -> ()
            n3265 = global write "Global display 3.vi" "TEMP RS 02-2"(w5884) -> ()
            n3266 = global write "Global display 3.vi" "TEMP RS 04-2"(w5880) -> ()
            n3267 = global write "Global display 3.vi" "TEMP RS 01-2"(w5886) -> ()
            n3268 = global write "Global display 3.vi" "TEMP RS 03-1"(w5883) -> ()
            n3269 = global write "Global display 3.vi" "TEMP RS 04-1"(w5881) -> ()
            n3270 = global write "Global display 3.vi" "TEMP RS 01-1"(w5887) -> ()
